vi "Maui.Config.WriteOwningClass.vi"(8 "error in (no error)":errorcluster, 10 "Owning Class":refnum<class>, 11 "Maui.Config in":refnum<class "Maui.Config.lvclass">) -> (0 "error out":errorcluster, 3 "Maui.Config out":refnum<class "Maui.Config.lvclass">)   [LabVIEW 2020, in "Maui.Config.lvclass"]
uses:
  Maui.Config.lvclass
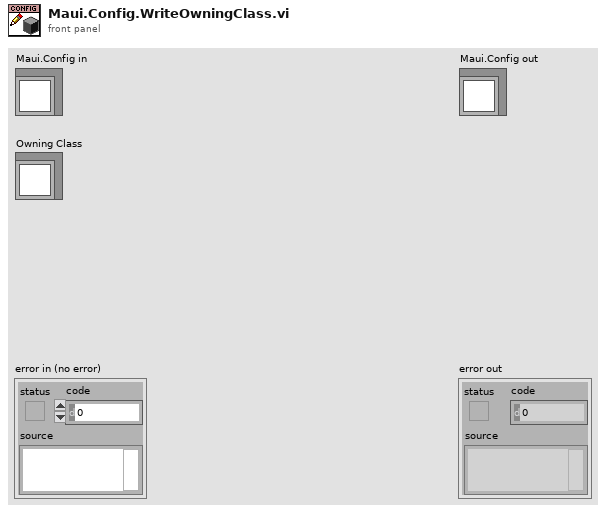
[diagram p1: front panel]
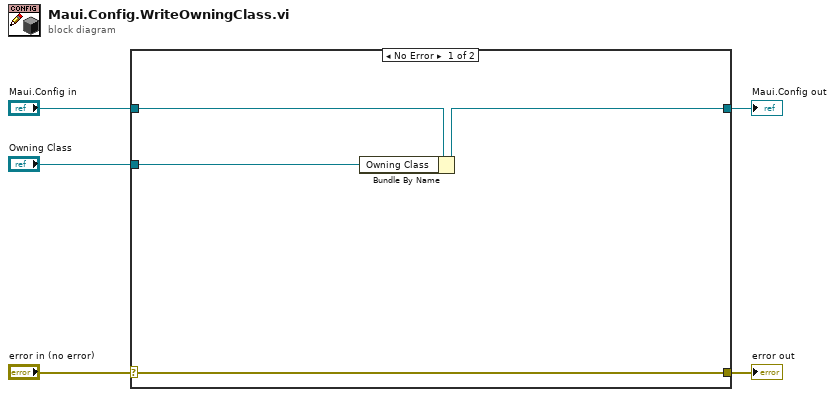
[diagram p0: block diagram]
diagram:
  n1 = case shown="No Error" "error in (no error)" {
    selector: "error in (no error)" -> [w9 w11]
    tunnel: [w9 w11] -> w4
    tunnel: [w8 w10] -> w2
    tunnel: "Maui.Config in" -> [w7 w10]
    tunnel: "Owning Class" -> [w6 _]
    frame No Error {
      n2 = Bundle By Name(cluster=w7, "Owning Class"=w6) -> (w8:refnum<class "Maui.Config.lvclass">)
    }
    frame Error {
    }
  }
  "error out" <- w4
  "Maui.Config out" <- w2
